vi "Move_Until_Home_from_anywhere.vi"(8 "error in":errorcluster, 11 "Machine In":refnum<visa-resource-name>) -> (0 "error out":errorcluster, 3 "Machine Out":refnum<visa-resource-name>)   [LabVIEW 2018]
panel:
  out "OUTPUT Z Coord":dbl
  out "OUTPUT X Coord":dbl
  out "OUTPUT Y Coord":dbl
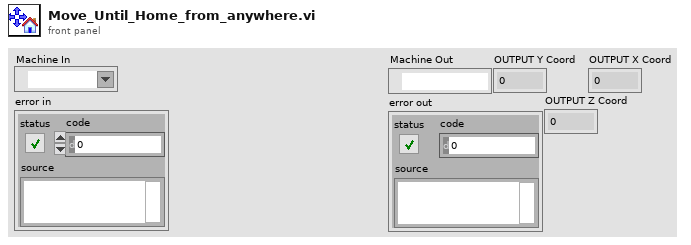
[diagram p1: front panel]
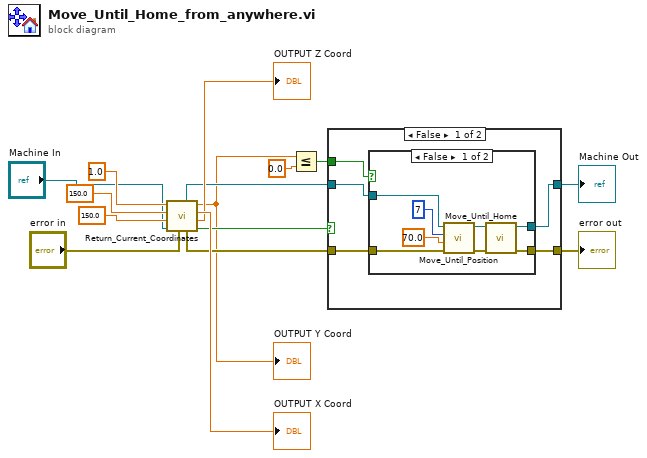
[diagram p0: block diagram]
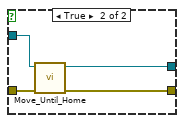
[diagram p2: hidden frame]
diagram:
  n1 = call "Return_Current_Coordinates.vi"("error in"="error in", "Machine In"="Machine In", "INPUT Z Coord"=150.0, "INPUT X Coord"=150.0, "INPUT Y Coord"=1.0) -> ("x = y?"=w8:bool, "OUTPUT Z Coord"=→"OUTPUT Z Coord":dbl, "OUTPUT X Coord"=→"OUTPUT X Coord":dbl, "OUTPUT Y Coord"=w4:dbl, "error out"=w7:errorcluster, "Machine Out"=w6:refnum<visa-resource-name>)  [unwired: 1 in]
  "OUTPUT Y Coord" <- w4
  n2 = Less Or Equal?(x=w4, y=0.0) -> (x <= y?=w2:bool)
  n3 = case shown="False" w8 {
    tunnel: w7 -> [w18 w34]
    tunnel: w6 -> [w19 w33]
    tunnel: [w17 w33] -> w5
    tunnel: w2 -> [w20 _]
    tunnel: [w16 w34] -> w1
    frame False {
      n4 = case shown="False" w20 {
        tunnel: w19 -> [w27 w32]
        tunnel: w18 -> [w28 w31]
        tunnel: [w24 w30] -> w17
        tunnel: [w21 w29] -> w16
        frame False {
          n5 = call "Move_Until_Position.vi"("error in (no error)"=w28, "Z-Position"=70.0, "index"=7, "VISA Refnum in"=w27) -> ("error out"=w22:errorcluster, "VISA Refnum out"=w23:refnum<visa-resource-name>)  [unwired: 6 in]
          n6 = call "Move_Until_Home.vi"("error in (no error)"=w22, "VISA Refnum in"=w23) -> ("error out"=w21:errorcluster, "VISA Refnum out"=w24:refnum<visa-resource-name>)  [unwired: 8 in]
        }
        frame True {
          n7 = call "Move_Until_Home.vi"("error in (no error)"=w31, "VISA Refnum in"=w32) -> ("error out"=w29:errorcluster, "VISA Refnum out"=w30:refnum<visa-resource-name>)  [unwired: 8 in]
        }
      }
    }
    frame True {
    }
  }
  "Machine Out" <- w5
  "error out" <- w1
